vi "laser_main.vi"() -> ()   [LabVIEW 2011]
panel:
  out "Alarm":i32
  out "Output":string
  in  "Custom command":string
  out "Back Reflection Monitor":i32
  out "appended array":bool[](array[boolean])
  in  "100percent":bool
  in  "75percent":bool
  in  "50percent":bool
  in  "25percent":bool
  in  "power 0":bool
  in  "Set Power":i32 max=2170
  out "Power":i32
  out "Current Power":u8(slide) scale=0.0..100.0
  out "max Q":i32
  out "error out":errorcluster
  in  "Laser COM PORT":refnum<visa-resource-name>="COM3"
  out "MachineState":string="init"
  in  "KEY":bool
  in  "stop":bool
  # "SET POWER"
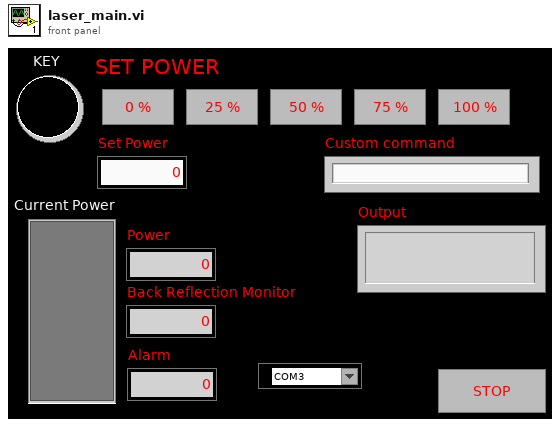
[diagram p1: front panel]
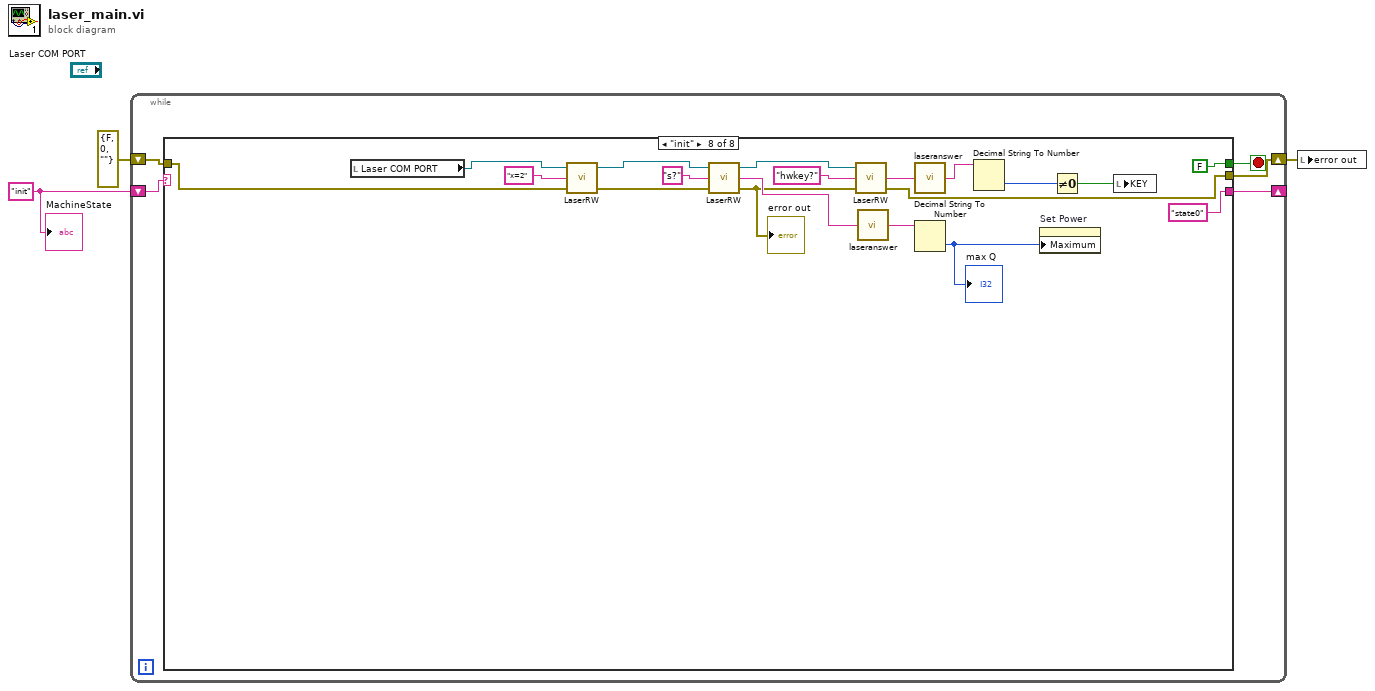
[diagram p0: block diagram]
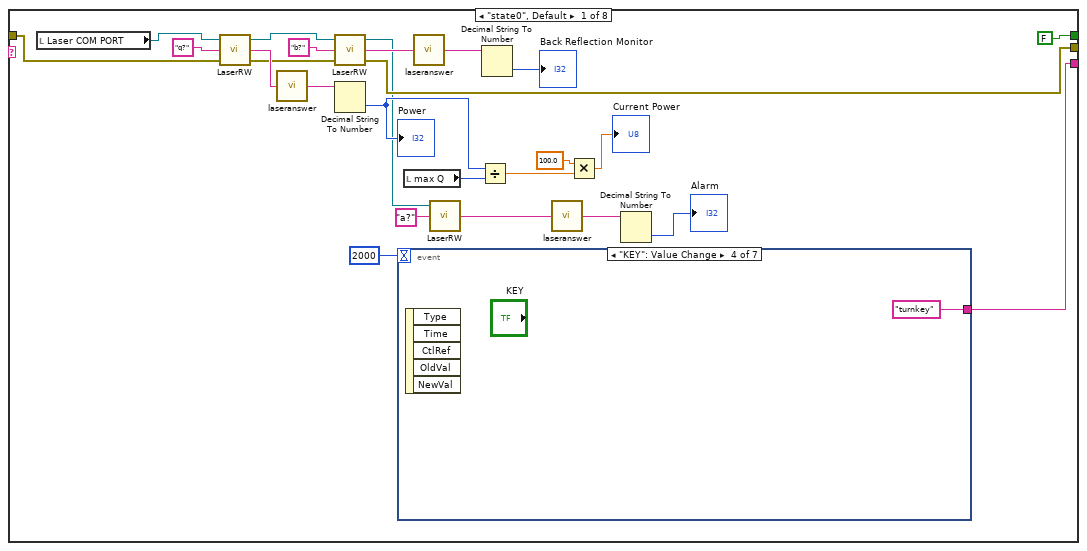
[diagram p2: hidden frame]
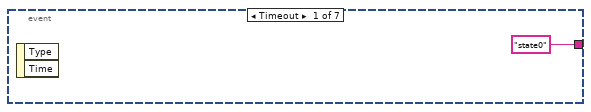
[diagram p3: hidden frame]
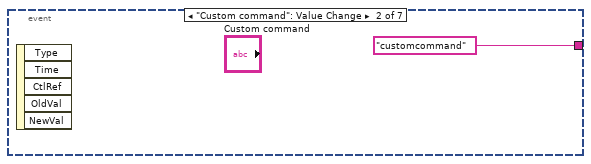
[diagram p4: hidden frame]
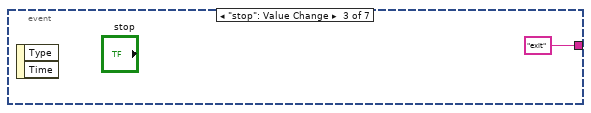
[diagram p5: hidden frame]
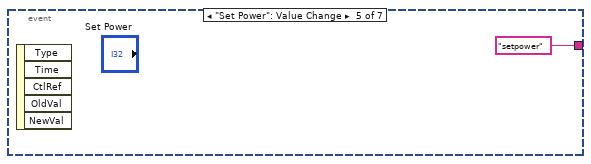
[diagram p6: hidden frame]
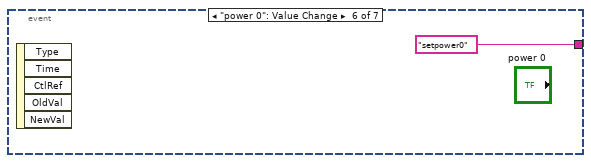
[diagram p7: hidden frame]
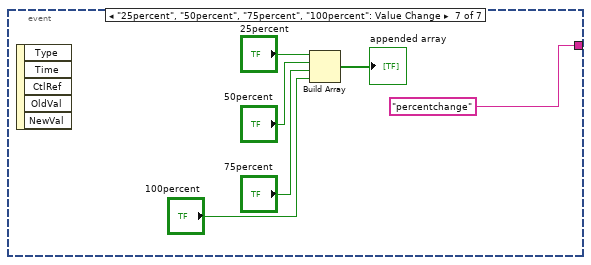
[diagram p8: hidden frame]
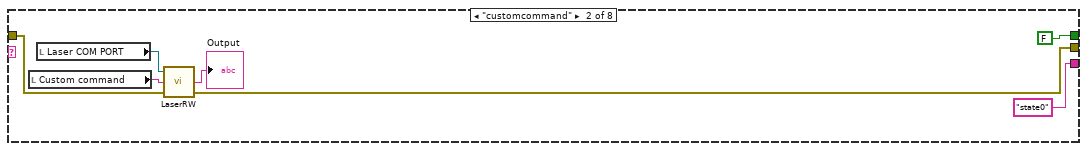
[diagram p9: hidden frame]
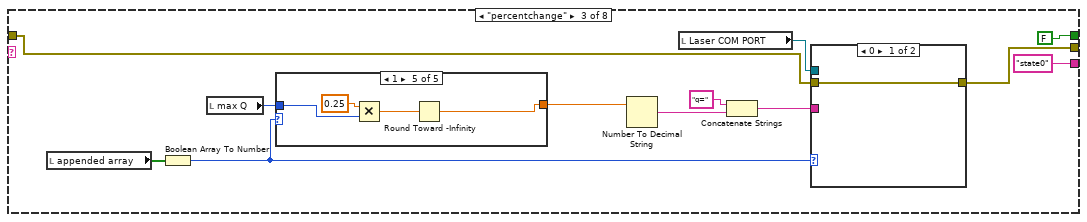
[diagram p10: hidden frame]
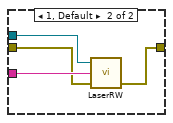
[diagram p11: hidden frame]
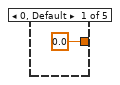
[diagram p12: hidden frame]
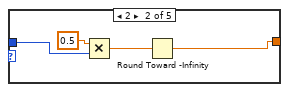
[diagram p13: hidden frame]
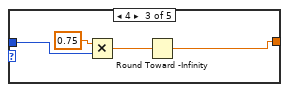
[diagram p14: hidden frame]
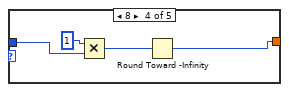
[diagram p15: hidden frame]
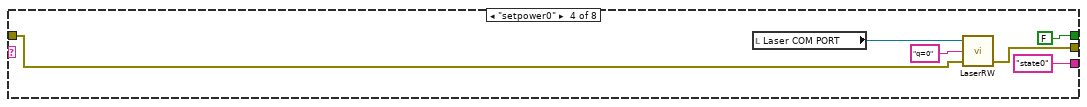
[diagram p16: hidden frame]
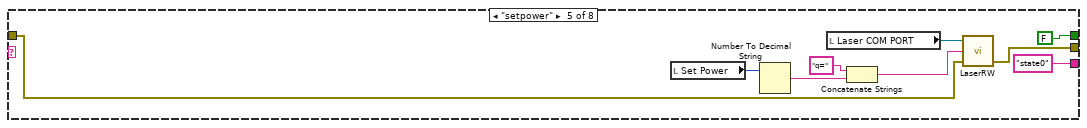
[diagram p17: hidden frame]
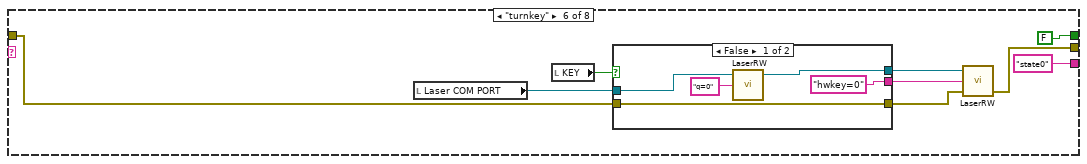
[diagram p18: hidden frame]
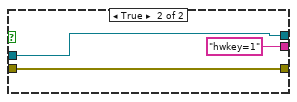
[diagram p19: hidden frame]
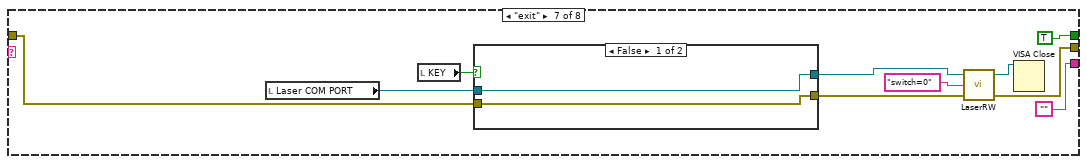
[diagram p20: hidden frame]
diagram:
  w3 = "init"
  n1 = while {
    shift-right: [w7] -> _
    shift-left: w3 -> [w8]
    shift-right: [w5] -> w2
    shift-left: errorcluster {"status"=FALSE, "code"=0, "source"=""} ("error out") -> [w4]
    stop <- w6 stop-if-true
    n2 = case shown="\"init\"" w8 {
      tunnel: [w33 "state0" "state0" "state0" "state0" "state0" "" "state0"] -> w7
      tunnel: [FALSE FALSE FALSE FALSE FALSE FALSE TRUE FALSE] -> w6
      tunnel: [w18 w50 w58 w89 w94 w103 w120 w141] -> w5
      tunnel: w4 -> [w31 w51 w57 w90 w101 w105 w124 w143]
      frame "state0", Default {
        n3 = local read "Laser COM PORT"() -> (w32:refnum<visa-resource-name>)
        n4 = call "LaserRW.vi"("error in (no error)"=w31, "buffer à écrire"="q?", "Nom de ressource VISA"=w32) -> ("error out"=w21:errorcluster, "buffer lu"=w29:string, "Nom de ressource VISA en sortie"=w22:refnum<visa-resource-name>)
        n5 = call "laseranswer.vi"("IN"=w29) -> ("Answer"=w28:string)
        n6 = call "LaserRW.vi"("error in (no error)"=w21, "buffer à écrire"="b?", "Nom de ressource VISA"=w22) -> ("error out"=w18:errorcluster, "buffer lu"=w19:string, "Nom de ressource VISA en sortie"=w13:refnum<visa-resource-name>)
        n7 = Decimal String To Number(string=w28) -> (number=w26:i32)  [unwired: 2 in, 1 out]
        "Power" <- w26
        n8 = event shown="[3] \"KEY\": Value Change" {
          selector: _ -> [_ _ _ _ _ _ _]
          dyn-events: _ -> [_ _ _ _ _ _ _]
          timeout: 2000 -> [_ _ _ _ _ _ _]
          tunnel: ["state0" "customcommand" "exit" "turnkey" "setpower" "setpower0" "percentchange"] -> w33
          event Timeout {
            n9 = event-data() -> ()  [unwired: 1 in, 2 out]
          }
          event "Custom command": Value Change {
            n10 = event-data() -> ()  [unwired: 1 in, 5 out]
          }
          event "stop": Value Change {
            n11 = event-data() -> ()  [unwired: 1 in, 2 out]
          }
          event "KEY": Value Change {
            n12 = event-data() -> ()  [unwired: 1 in, 5 out]
          }
          event "Set Power": Value Change {
            n13 = event-data() -> ()  [unwired: 1 in, 5 out]
          }
          event "power 0": Value Change {
            n14 = event-data() -> ()  [unwired: 1 in, 5 out]
          }
          event "25percent", "50percent", "75percent", "100percent": Value Change {
            n15 = event-data() -> ()  [unwired: 1 in, 5 out]
            n16 = Build Array("25percent", "50percent", "75percent", "100percent") -> (→"appended array":bool[])
          }
        }
        n17 = local read "max Q"() -> (w27:i32)
        n18 = call "laseranswer.vi"("IN"=w19) -> ("Answer"=w17:string)
        n19 = call "LaserRW.vi"("buffer à écrire"="a?", "Nom de ressource VISA"=w13) -> ("buffer lu"=w14:string)  [unwired: 1 in, 2 out]
        n20 = Divide(x=w26, y=w27) -> (x/y=w25:dbl)
        n21 = Decimal String To Number(string=w17) -> (number=→"Back Reflection Monitor":i32)  [unwired: 2 in, 1 out]
        n22 = call "laseranswer.vi"("IN"=w14) -> ("Answer"=w12:string)
        n23 = Multiply(x=100.0, y=w25) -> (x*y=→"Current Power":dbl)
        n24 = Decimal String To Number(string=w12) -> (number=→"Alarm":i32)  [unwired: 2 in, 1 out]
      }
      frame "customcommand" {
        n25 = local read "Custom command"() -> (w52:string)
        n26 = local read "Laser COM PORT"() -> (w48:refnum<visa-resource-name>)
        n27 = call "LaserRW.vi"("error in (no error)"=w51, "buffer à écrire"=w52, "Nom de ressource VISA"=w48) -> ("error out"=w50:errorcluster, "buffer lu"=→"Output":string)  [unwired: 1 out]
      }
      frame "percentchange" {
        n28 = local read "appended array"() -> (w63:bool[])
        n29 = Boolean Array To Number(Boolean array=w63) -> (number=w54:u32)
        n30 = local read "max Q"() -> (w62:i32)
        n31 = case shown="1" w54 {
          tunnel: w62 -> [_ w71 w75 w80 w85]
          tunnel: [0.0 w72 w76 w79 w83] -> w55
          frame 0, Default {
          }
          frame 2 {
            n32 = Multiply(x=0.5, y=w71) -> (x*y=w73:dbl)
            n33 = Round Toward -Infinity(1:w73) -> (0:w72:dbl)
          }
          frame 4 {
            n34 = Multiply(x=0.75, y=w75) -> (x*y=w77:dbl)
            n35 = Round Toward -Infinity(1:w77) -> (0:w76:dbl)
          }
          frame 8 {
            n36 = Multiply(x=1, y=w80) -> (x*y=w81:i32)
            n37 = Round Toward -Infinity(1:w81) -> (0:w79:i32)
          }
          frame 1 {
            n38 = Multiply(x=0.25, y=w85) -> (x*y=w84:dbl)
            n39 = Round Toward -Infinity(1:w84) -> (0:w83:dbl)
          }
        }
        n40 = Number To Decimal String(number=w55) -> (decimal integer string=w61:string)  [unwired: 1 in]
        n41 = local read "Laser COM PORT"() -> (w56:refnum<visa-resource-name>)
        n42 = Concatenate Strings("q=" ("string"), w61) -> (w59:string)
        n43 = case shown="0" w54 {
          tunnel: w59 -> [_ w69]
          tunnel: [w65 w68] -> w58
          tunnel: w57 -> [w65 w67]
          tunnel: w56 -> [_ w66]
          frame 0 {
          }
          frame 1, Default {
            n44 = call "LaserRW.vi"("error in (no error)"=w67, "buffer à écrire"=w69, "Nom de ressource VISA"=w66) -> ("error out"=w68:errorcluster)  [unwired: 2 out]
          }
        }
      }
      frame "setpower0" {
        n45 = local read "Laser COM PORT"() -> (w91:refnum<visa-resource-name>)
        n46 = call "LaserRW.vi"("error in (no error)"=w90, "buffer à écrire"="q=0", "Nom de ressource VISA"=w91) -> ("error out"=w89:errorcluster)  [unwired: 2 out]
      }
      frame "setpower" {
        n47 = local read "Set Power"() -> (w100:i32)
        n48 = Number To Decimal String(number=w100) -> (decimal integer string=w99:string)  [unwired: 1 in]
        n49 = local read "Laser COM PORT"() -> (w96:refnum<visa-resource-name>)
        n50 = Concatenate Strings("q=" ("string"), w99) -> (w97:string)
        n51 = call "LaserRW.vi"("error in (no error)"=w101, "buffer à écrire"=w97, "Nom de ressource VISA"=w96) -> ("error out"=w94:errorcluster)  [unwired: 2 out]
      }
      frame "turnkey" {
        n52 = local read "Laser COM PORT"() -> (w107:refnum<visa-resource-name>)
        n53 = local read "KEY"() -> (w109:bool)
        n54 = case shown="False" w109 {
          tunnel: ["hwkey=0" "hwkey=1"] -> w108
          tunnel: w107 -> [w115 w117]
          tunnel: [w113 w117] -> w106
          tunnel: w105 -> [w112 w116]
          tunnel: [w112 w116] -> w104
          frame False {
            n55 = call "LaserRW.vi"("buffer à écrire"="q=0", "Nom de ressource VISA"=w115) -> ("Nom de ressource VISA en sortie"=w113:refnum<visa-resource-name>)  [unwired: 1 in, 2 out]
          }
          frame True {
          }
        }
        n56 = call "LaserRW.vi"("error in (no error)"=w104, "buffer à écrire"=w108, "Nom de ressource VISA"=w106) -> ("error out"=w103:errorcluster)  [unwired: 2 out]
      }
      frame "exit" {
        n57 = local read "Laser COM PORT"() -> (w126:refnum<visa-resource-name>)
        n58 = local read "KEY"() -> (w125:bool)
        n59 = case shown="False" w125 {
          tunnel: w126 -> [w129 w138]
          tunnel: w124 -> [w130 w134]
          tunnel: [w130 w132] -> w123
          tunnel: [w129 w131] -> w122
          frame False {
          }
          frame True {
            n60 = call "LaserRW.vi"("error in (no error)"=w134, "buffer à écrire"="q=0", "Nom de ressource VISA"=w138) -> ("error out"=w133:errorcluster, "Nom de ressource VISA en sortie"=w135:refnum<visa-resource-name>)  [unwired: 1 out]
            n61 = call "LaserRW.vi"("error in (no error)"=w133, "buffer à écrire"="hwkey=0", "Nom de ressource VISA"=w135) -> ("error out"=w132:errorcluster, "Nom de ressource VISA en sortie"=w131:refnum<visa-resource-name>)  [unwired: 1 out]
          }
        }
        n62 = call "LaserRW.vi"("error in (no error)"=w123, "buffer à écrire"="switch=0", "Nom de ressource VISA"=w122) -> ("error out"=w120:errorcluster, "Nom de ressource VISA en sortie"=w119:refnum<visa-resource-name>)  [unwired: 1 out]
        n63 = VISA Close(VISA resource name=w119) -> ()  [unwired: 1 in, 1 out]
      }
      frame "init" {
        n64 = local read "Laser COM PORT"() -> (w140:refnum<visa-resource-name>)
        n65 = call "LaserRW.vi"("error in (no error)"=w143, "buffer à écrire"="x=2", "Nom de ressource VISA"=w140) -> ("error out"=w142:errorcluster, "Nom de ressource VISA en sortie"=w139:refnum<visa-resource-name>)  [unwired: 1 out]
        n66 = call "LaserRW.vi"("error in (no error)"=w142, "buffer à écrire"="s?", "Nom de ressource VISA"=w139) -> ("error out"=w144:errorcluster, "buffer lu"=w155:string, "Nom de ressource VISA en sortie"=w151:refnum<visa-resource-name>)
        "error out" <- w144
        n67 = call "LaserRW.vi"("error in (no error)"=w144, "buffer à écrire"="hwkey?", "Nom de ressource VISA"=w151) -> ("error out"=w141:errorcluster, "buffer lu"=w150:string)  [unwired: 1 out]
        n68 = call "laseranswer.vi"("IN"=w155) -> ("Answer"=w154:string)
        n69 = call "laseranswer.vi"("IN"=w150) -> ("Answer"=w148:string)
        n70 = Decimal String To Number(string=w154) -> (number=w153:i32)  [unwired: 2 in, 1 out]
        "max Q" <- w153
        n71 = Decimal String To Number(string=w148) -> (number=w147:i32)  [unwired: 2 in, 1 out]
        n72 = property on="Set Power" class="DigNum (strict)"("Maximum"=w153) -> ()  [unwired: 2 in, 2 out]
        n73 = Not Equal To 0?(x=w147) -> (x != 0?=w146:bool)
        n74 = local write "KEY"(w146) -> ()
      }
    }
  }
  n75 = local write "error out"(w2) -> ()
  "MachineState" <- w3
